vi "Scanner Queue - Create.vi"(8 "error in":errorcluster, 11 "VI In":refnum<vi>) -> (0 "error out":errorcluster)   [LabVIEW 2024, in "Session Scanner.lvlib"]
uses:
  Session Scanner.lvlib
  Support/General Type Defs/FGV States.ctl
  Support/General Type Defs/General Type Definitions.lvlib
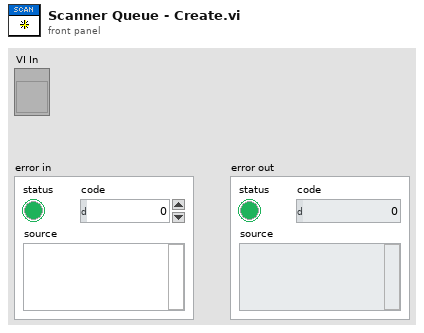
[diagram p1: front panel]
types:
  T1 = typedef "General Type Definitions.lvlib/FGV States.ctl" = enum16{"Create", "Get", "Destroy"}
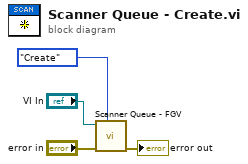
[diagram p0: block diagram]
diagram:
  n1 = call "Scanner Queue - FGV.vi"("FGV States"=FGV_States."Create", "error in"="error in", "VI In"="VI In") -> ("error out"=→"error out":errorcluster)  [unwired: 7 in, 1 out]
